vi "SendSetValue.vi"(8 "error in (no error)":errorcluster, 9 "Data":variant, 10 "PVName":string, 11 "PVConnections":refnum<class "PVConnection.lvclass">[](array[class])) -> (0 "error out":errorcluster, 3 "PVConnection out":refnum<class "PVConnection.lvclass">)   [LabVIEW 2014, in "CS++ScopeGui.lvlib" / "CS++ScopeGui.lvclass"]
uses:
  CS++ScopeGui.lvclass
  CSPP_Core/Classes/CS++ProcessVariables/PVConnection/PVConnection.lvclass
  CSPP_Core/Classes/CS++ProcessVariables/PVConnection/PVConnection.lvclass/PVConnection.ctl
  CSPP_Core/Classes/CS++ProcessVariables/ProcessVariable/PV.lvclass/PV.ctl
  CSPP_Core/Classes/CS++ProcessVariables/ProcessVariable/PV.lvclass
panel:
  out "Found?":bool
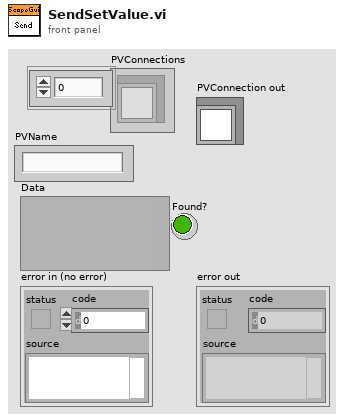
[diagram p1: front panel]
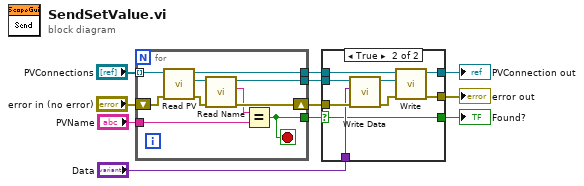
[diagram p0: block diagram]
diagram:
  n1 = for {
    tunnel: [w21] -> w11
    tunnel: [w17] -> w9
    shift-right: [w16] -> w10
    shift-left: "error in (no error)" -> [w20]
    tunnel: "PVConnections" -> [w19] mode=indexing
    tunnel: "PVName" -> [w13]
    tunnel: [w12] -> w2
    stop <- w12 stop-if-true
    n2 = call "Read PV.vi"("error in (no error)"=w20, "PVConnection in"=w19) -> ("error out"=w15:errorcluster, "PV"=w18:refnum<class "PV.lvclass">, "PVConnection out"=w21:refnum<class "PVConnection.lvclass">)  [unwired: 7 in]
    n3 = call "Read Name.vi"("error in (no error)"=w15, "PV in"=w18) -> ("error out"=w16:errorcluster, "Name"=w14:string, "PV out"=w17:refnum<class "PV.lvclass">)  [unwired: 7 in]
    n4 = Equal?(x=w14, y=w13) -> (x = y?=w12:bool)
  }
  n5 = case shown="True" w2 {
    selector: w2 -> [w23 w25]
    tunnel: w11 -> [w24 w33]
    tunnel: w10 -> [w22 w30]
    tunnel: w9 -> [_ w29]
    tunnel: "Data" -> [_ w28]
    tunnel: [w22 w27] -> w6
    tunnel: [w24 w26] -> w5
    tunnel: [w23 w25] -> w1
    frame False {
    }
    frame True {
      n6 = call "Write Data.vi"("error in (no error)"=w30, "Data"=w28, "PV in"=w29) -> ("error out"=w32:errorcluster, "PV out"=w31:refnum<class "PV.lvclass">)  [unwired: 7 in]
      n7 = call "Write.vi"("error in (no error)"=w32, "PV"=w31, "PVConnection in"=w33) -> ("error out"=w27:errorcluster, "PVConnection out"=w26:refnum<class "PVConnection.lvclass">)  [unwired: 7 in]
    }
  }
  "error out" <- w6
  "PVConnection out" <- w5
  "Found?" <- w1
